vi "Get_devices_information.vi"(8 "error in (no error)":errorcluster, 11 "Toolbox in":refnum<class "Toolbox.lvclass">) -> (0 "error out":errorcluster, 2 "devices_found":i32, 3 "Toolbox out":refnum<class "Toolbox.lvclass">)   [LabVIEW 2014, in "Driver_interaction.lvlib" / "Toolbox.lvclass"]
uses:
  Toolbox.lvclass
  _Driver_interaction/_Driver_interaction.lvclass/_Driver_interaction.ctl
  Toolbox.lvclass/Toolbox.ctl
  Vendor/lib 2p0/types/interface_type.ctl
  _Driver_interaction/_Driver_interaction.lvclass
  Vendor/lib 2p0/FTS 2p0.lvlib
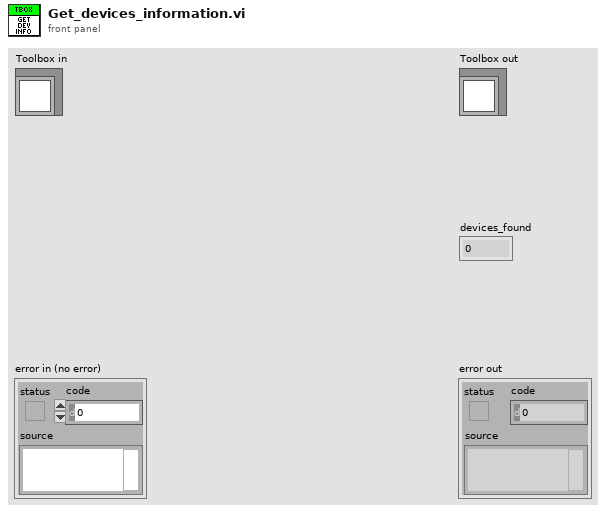
[diagram p1: front panel]
types:
  T1 = typedef "FTS 2p0.lvlib/interface_type.ctl" = string
  T2 = typedef "Driver_interaction.lvlib/_Driver_interaction.lvclass/Interface_type.ctl" = string
  T3 = typedef "Driver_interaction.lvlib/Toolbox.lvclass/Toolbox_session.ctl" = cluster{"client handle":T4, "URL out":string, "universe_id":i32, "devices_id":i32[]}
  T4 = typedef "LabVIEWHTTPClient.lvlib/ClientHandle.ctl" = refnum<k1>
  T5 = cluster{"device_id":i32, "device_name":string, "interface_type":T1, "manufacturer":string, "revision":string, "state":string, "unique_id_string":string}[]
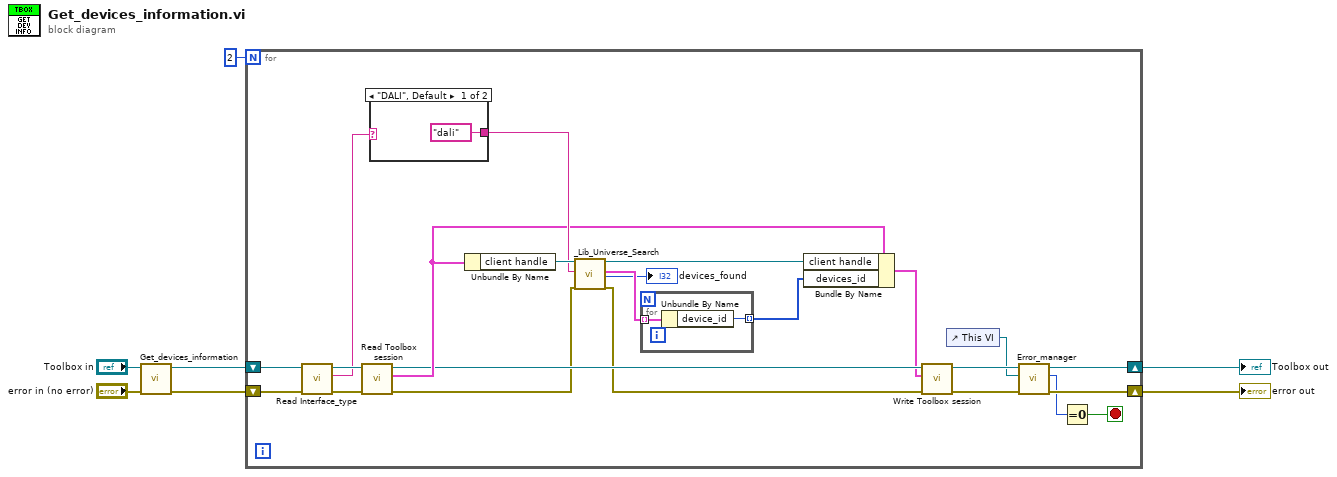
[diagram p0: block diagram]
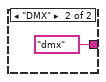
[diagram p2: hidden frame]
diagram:
  n1 = call-parent "Get_devices_information.vi"("error in (no error)"="error in (no error)", "_Driver_interaction in"="Toolbox in") -> ("error out"=w3:errorcluster, "_Driver_interaction out"=w2:refnum<class "Toolbox.lvclass">)  [unwired: 7 in, 1 out]
  n2 = for {
    N: 2 -> [_]
    shift-right: [w13] -> w4
    shift-left: w3 -> [w29]
    shift-right: [w14] -> w5
    shift-left: w2 -> [w28]
    stop <- w11 stop-if-true
    n3 = call "Read Interface_type.vi"("error in (no error)"=w29, "_Driver_interaction in"=w28) -> ("error out"=w26:errorcluster, "Interface_type"=w25:T2, "_Driver_interaction out"=w27:refnum<class "Toolbox.lvclass">)  [unwired: 7 in]
    n4 = call "Read Toolbox session.vi"("error in (no error)"=w26, "Toolbox in"=w27) -> ("error out"=w9:errorcluster, "Toolbox session"=w23:T3, "Toolbox out"=w18:refnum<class "Toolbox.lvclass">)  [unwired: 7 in]
    n5 = case shown="\"DALI\", Default" w25 {
      tunnel: [T1 "dali" ("params.interface_type") T1 "dmx" ("params.interface_type")] -> w24
      frame "DALI", Default {
      }
      frame "DMX" {
      }
    }
    n6 = Unbundle By Name(w23) -> ("client handle"=w30:T4)
    n7 = call "_Lib_Universe_Search.vi"("client handle"=w30, "params.interface_type"=w24, "error in (no error)"=w9) -> ("client handle out"=w22:T4, "result"=w21:T5, "#devices"=→"devices_found":i32, "error out"=w8:errorcluster)  [unwired: 12 in, 1 out]
    n8 = for {
      tunnel: w21 -> [w32] mode=indexing
      tunnel: [w31] -> w19 mode=indexing
      n9 = Unbundle By Name(w32) -> ("device_id"=w31:i32)
    }
    n10 = Bundle By Name(cluster=w23, "client handle"=w22, "devices_id"=w19) -> (w17:T3)
    n11 = call "Write Toolbox session.vi"("error in (no error)"=w8, "Toolbox session"=w17, "Toolbox in"=w18) -> ("error out"=w16:errorcluster, "Toolbox out"=w15:refnum<class "Toolbox.lvclass">)  [unwired: 7 in]
    n12 = control-ref of="This VI"() -> (w10:refnum<vi>)
    n13 = call-dynamic "Error_manager.vi"("error in (no error)"=w16, "Caller VI"=w10, "Toolbox in"=w15) -> ("error out"=w13:errorcluster, "code"=w12:i32, "Toolbox out"=w14:refnum<class "Toolbox.lvclass">)  [unwired: 4 in, 2 out]
    n14 = Equal To 0?(x=w12) -> (x = 0?=w11:bool)
  }
  "error out" <- w4
  "Toolbox out" <- w5
